vi "MIDI command to application state.vi"(9 "MIDI Command":T1={"Device"=enum."Pads", "Parameter 1"=0, "Parameter 2"=0}, 11 "Note Queue":refnum<queue>) -> ()   [LabVIEW 2015]
uses:
  Controls/playback state.ctl
  Controls/Application Data.vi
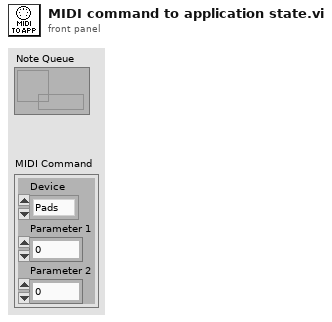
[diagram p1: front panel]
types:
  T1 = cluster{"Device":enum16{"Keys", "Controls", "Pads"}, "Parameter 1":u8, "Parameter 2":u8}
  T2 = typedef "playback state.ctl" = enum16{"Load File", "Save File", "Play", "Record", "Stop", "Rewind"}
  T3 = typedef "Track Controls.ctl" = cluster{"Track 0":T4, "Track 1":T4, "Track 2":T4, "Track 3":T4}
  T4 = typedef "Track Volume Settings.ctl" = cluster{"Volume":dbl, "Pan":dbl, "Record":bool, "FX":bool}
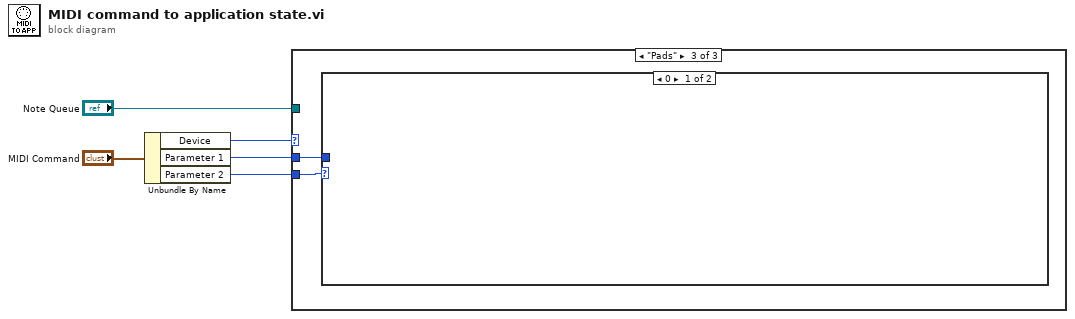
[diagram p0: block diagram]
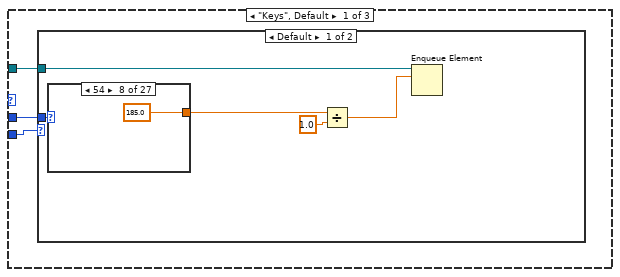
[diagram p2: hidden frame]
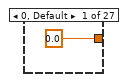
[diagram p3: hidden frame]
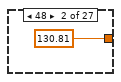
[diagram p4: hidden frame]
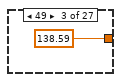
[diagram p5: hidden frame]
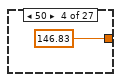
[diagram p6: hidden frame]
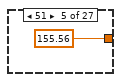
[diagram p7: hidden frame]
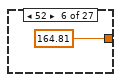
[diagram p8: hidden frame]
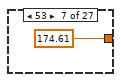
[diagram p9: hidden frame]
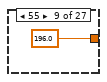
[diagram p10: hidden frame]
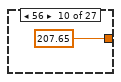
[diagram p11: hidden frame]
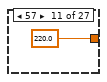
[diagram p12: hidden frame]
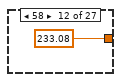
[diagram p13: hidden frame]
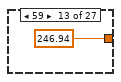
[diagram p14: hidden frame]
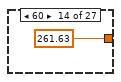
[diagram p15: hidden frame]
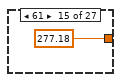
[diagram p16: hidden frame]
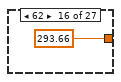
[diagram p17: hidden frame]
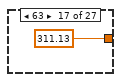
[diagram p18: hidden frame]
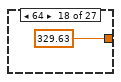
[diagram p19: hidden frame]
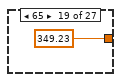
[diagram p20: hidden frame]
diagram:
  n1 = Unbundle By Name("MIDI Command") -> ("Device"=w4:enum16{"Keys", "Controls", "Pads"}, "Parameter 1"=w3:u8, "Parameter 2"=w1:u8)
  n2 = case shown="\"Pads\"" w4 {
    tunnel: w3 -> [w8 w42 w101]
    tunnel: "Note Queue" -> [w7 _ _]
    tunnel: w1 -> [w6 w41 w100]
    frame "Keys", Default {
      n3 = case shown="Default" w6 {
        tunnel: w8 -> [w10 _]
        tunnel: w7 -> [w9 _]
        frame Default {
          n4 = case shown="54" w10 {
            tunnel: [0.0 130.81 138.59 146.83 155.56 164.81 174.61 185.0 196.0 207.65 220.0 233.08 246.94 261.63 277.18 293.66 311.13 329.63 349.23 369.99 392.0 415.3 440.0 466.16 493.88 523.25 554.37] -> w13
            frame 0, Default {
            }
            frame 48 {
            }
            frame 49 {
            }
            frame 50 {
            }
            frame 51 {
            }
            frame 52 {
            }
            frame 53 {
            }
            frame 54 {
            }
            frame 55 {
            }
            frame 56 {
            }
            frame 57 {
            }
            frame 58 {
            }
            frame 59 {
            }
            frame 60 {
            }
            frame 61 {
            }
            frame 62 {
            }
            frame 63 {
            }
            frame 64 {
            }
            frame 65 {
            }
            frame 66 {
            }
            frame 67 {
            }
            frame 68 {
            }
            frame 69 {
            }
            frame 70 {
            }
            frame 71 {
            }
            frame 72 {
            }
            frame 73 {
            }
          }
          n5 = Divide(x=w13, y=1.0) -> (x/y=w11:dbl)
          n6 = Enqueue Element(queue=w9, element=w11) -> ()  [unwired: 2 in, 3 out]
        }
        frame 0 {
        }
      }
    }
    frame "Controls" {
      n7 = case shown="10" w42 {
        tunnel: w41 -> [_ _ w47 _ _ w54 w60 w66 w72 w78 w84 w90 w96 _ _]
        frame 24 {
          n8 = global write "Application Data.vi" "Playback State"(playback_state."Play" ("Next State")) -> ()
        }
        frame 0, Default {
        }
        frame 1 {
          n9 = To Double Precision Float(number=w47) -> (double precision float=w46:dbl)
          n10 = Multiply(x=w46, y=132104.0) -> (x*y=w45:dbl)
          n11 = To Unsigned Long Integer(number=w45) -> (unsigned 32bit integer=w44:u32)
          n12 = global write "Application Data.vi" "Delay"(w44) -> ()
        }
        frame 25 {
          n13 = global write "Application Data.vi" "Playback State"(playback_state."Record" ("Next State")) -> ()
        }
        frame 20 {
          n14 = call "reset.vi"() -> ()  [unwired: 11 in, 1 out]
        }
        frame 71 {
          n15 = Divide(x=w54, y=12.7) -> (x/y=w52:dbl)
          n16 = global read "Application Data.vi" "Track Controls"() -> (w51:T3)
          n17 = in-place {
            in-place-border: w52 -> [w55]
            n18 = in-place-cluster #1(w51) -> ()  [unwired: 1 out]
            n19 = in-place-cluster #1("Track 0.Volume"=w55) -> (w50:T3)
          }
          n20 = global write "Application Data.vi" "Track Controls"(w50) -> ()
        }
        frame 91 {
          n21 = Divide(x=w60, y=127.0) -> (x/y=w58:dbl)
          n22 = global read "Application Data.vi" "Track Controls"() -> (w57:T3)
          n23 = in-place {
            in-place-border: w58 -> [w61]
            n24 = in-place-cluster #2(w57) -> ()  [unwired: 1 out]
            n25 = in-place-cluster #2("Track 0.Pan"=w61) -> (w56:T3)
          }
          n26 = global write "Application Data.vi" "Track Controls"(w56) -> ()
        }
        frame 74 {
          n27 = Divide(x=w66, y=12.7) -> (x/y=w64:dbl)
          n28 = global read "Application Data.vi" "Track Controls"() -> (w63:T3)
          n29 = in-place {
            in-place-border: w64 -> [w67]
            n30 = in-place-cluster #3(w63) -> ()  [unwired: 1 out]
            n31 = in-place-cluster #3("Track 1.Volume"=w67) -> (w62:T3)
          }
          n32 = global write "Application Data.vi" "Track Controls"(w62) -> ()
        }
        frame 93 {
          n33 = Divide(x=w72, y=127.0) -> (x/y=w70:dbl)
          n34 = global read "Application Data.vi" "Track Controls"() -> (w69:T3)
          n35 = in-place {
            in-place-border: w70 -> [w73]
            n36 = in-place-cluster #4(w69) -> ()  [unwired: 1 out]
            n37 = in-place-cluster #4("Track 1.Pan"=w73) -> (w68:T3)
          }
          n38 = global write "Application Data.vi" "Track Controls"(w68) -> ()
        }
        frame 84 {
          n39 = Divide(x=w78, y=12.7) -> (x/y=w76:dbl)
          n40 = global read "Application Data.vi" "Track Controls"() -> (w75:T3)
          n41 = in-place {
            in-place-border: w76 -> [w79]
            n42 = in-place-cluster #5(w75) -> ()  [unwired: 1 out]
            n43 = in-place-cluster #5("Track 2.Volume"=w79) -> (w74:T3)
          }
          n44 = global write "Application Data.vi" "Track Controls"(w74) -> ()
        }
        frame 5 {
          n45 = Divide(x=w84, y=127.0) -> (x/y=w82:dbl)
          n46 = global read "Application Data.vi" "Track Controls"() -> (w81:T3)
          n47 = in-place {
            in-place-border: w82 -> [w85]
            n48 = in-place-cluster #6(w81) -> ()  [unwired: 1 out]
            n49 = in-place-cluster #6("Track 2.Pan"=w85) -> (w80:T3)
          }
          n50 = global write "Application Data.vi" "Track Controls"(w80) -> ()
        }
        frame 7 {
          n51 = Divide(x=w90, y=12.7) -> (x/y=w88:dbl)
          n52 = global read "Application Data.vi" "Track Controls"() -> (w87:T3)
          n53 = in-place {
            in-place-border: w88 -> [w91]
            n54 = in-place-cluster #7(w87) -> ()  [unwired: 1 out]
            n55 = in-place-cluster #7("Track 3.Volume"=w91) -> (w86:T3)
          }
          n56 = global write "Application Data.vi" "Track Controls"(w86) -> ()
        }
        frame 10 {
          n57 = Divide(x=w96, y=127.0) -> (x/y=w94:dbl)
          n58 = global read "Application Data.vi" "Track Controls"() -> (w93:T3)
          n59 = in-place {
            in-place-border: w94 -> [w97]
            n60 = in-place-cluster #8(w93) -> ()  [unwired: 1 out]
            n61 = in-place-cluster #8("Track 3.Pan"=w97) -> (w92:T3)
          }
          n62 = global write "Application Data.vi" "Track Controls"(w92) -> ()
        }
        frame 23 {
          n63 = global write "Application Data.vi" "Playback State"(playback_state."Stop" ("Next State")) -> ()
        }
        frame 21 {
          n64 = global write "Application Data.vi" "Playback State"(playback_state."Rewind" ("Next State")) -> ()
        }
      }
    }
    frame "Pads" {
      n65 = case shown="0" w100 {
        tunnel: w101 -> [_ w102]
        frame 0 {
        }
        frame Default {
          n66 = case shown="50" w102 {
            frame 0, Default {
            }
            frame 50 {
              n67 = global read "Application Data.vi" "Track Controls"() -> (w104:T3)
              n68 = in-place {
                n69 = in-place-cluster #9(w104) -> ("Track 0.Record"=w106:bool)
                n70 = Not(x=w106) -> (.not. x?=w105:bool)
                n71 = in-place-cluster #9("Track 0.Record"=w105) -> (w103:T3)
              }
              n72 = global write "Application Data.vi" "Track Controls"(w103) -> ()
            }
            frame 45 {
              n73 = global read "Application Data.vi" "Track Controls"() -> (w108:T3)
              n74 = in-place {
                n75 = in-place-cluster #10(w108) -> ("Track 1.Record"=w110:bool)
                n76 = Not(x=w110) -> (.not. x?=w109:bool)
                n77 = in-place-cluster #10("Track 1.Record"=w109) -> (w107:T3)
              }
              n78 = global write "Application Data.vi" "Track Controls"(w107) -> ()
            }
            frame 51 {
              n79 = global read "Application Data.vi" "Track Controls"() -> (w112:T3)
              n80 = in-place {
                n81 = in-place-cluster #11(w112) -> ("Track 2.Record"=w114:bool)
                n82 = Not(x=w114) -> (.not. x?=w113:bool)
                n83 = in-place-cluster #11("Track 2.Record"=w113) -> (w111:T3)
              }
              n84 = global write "Application Data.vi" "Track Controls"(w111) -> ()
            }
            frame 49 {
              n85 = global read "Application Data.vi" "Track Controls"() -> (w116:T3)
              n86 = in-place {
                n87 = in-place-cluster #12(w116) -> ("Track 3.Record"=w118:bool)
                n88 = Not(x=w118) -> (.not. x?=w117:bool)
                n89 = in-place-cluster #12("Track 3.Record"=w117) -> (w115:T3)
              }
              n90 = global write "Application Data.vi" "Track Controls"(w115) -> ()
            }
            frame 36 {
              n91 = global read "Application Data.vi" "Track Controls"() -> (w120:T3)
              n92 = in-place {
                n93 = in-place-cluster #13(w120) -> ("Track 0.FX"=w122:bool)
                n94 = Not(x=w122) -> (.not. x?=w121:bool)
                n95 = in-place-cluster #13("Track 0.FX"=w121) -> (w119:T3)
              }
              n96 = global write "Application Data.vi" "Track Controls"(w119) -> ()
            }
            frame 38 {
              n97 = global read "Application Data.vi" "Track Controls"() -> (w124:T3)
              n98 = in-place {
                n99 = in-place-cluster #14(w124) -> ("Track 1.FX"=w126:bool)
                n100 = Not(x=w126) -> (.not. x?=w125:bool)
                n101 = in-place-cluster #14("Track 1.FX"=w125) -> (w123:T3)
              }
              n102 = global write "Application Data.vi" "Track Controls"(w123) -> ()
            }
            frame 46 {
              n103 = global read "Application Data.vi" "Track Controls"() -> (w128:T3)
              n104 = in-place {
                n105 = in-place-cluster #15(w128) -> ("Track 2.FX"=w130:bool)
                n106 = Not(x=w130) -> (.not. x?=w129:bool)
                n107 = in-place-cluster #15("Track 2.FX"=w129) -> (w127:T3)
              }
              n108 = global write "Application Data.vi" "Track Controls"(w127) -> ()
            }
            frame 42 {
              n109 = global read "Application Data.vi" "Track Controls"() -> (w132:T3)
              n110 = in-place {
                n111 = in-place-cluster #16(w132) -> ("Track 3.FX"=w134:bool)
                n112 = Not(x=w134) -> (.not. x?=w133:bool)
                n113 = in-place-cluster #16("Track 3.FX"=w133) -> (w131:T3)
              }
              n114 = global write "Application Data.vi" "Track Controls"(w131) -> ()
            }
          }
        }
      }
    }
  }
